vi "Get Menu Bottom Position.vi"(8 "error in (no error)":errorcluster, 11 "MenuButton in":refnum<class "MenuButton.lvclass">) -> (0 "error out":errorcluster, 2 "Menu Bottom Position":u32, 3 "MenuButton out":refnum<class "MenuButton.lvclass">)   [LabVIEW 2017, in "MenuButtons.lvlib" / "MenuButton.lvclass"]
uses:
  MenuButton.lvclass
  MenuButton.lvclass/MenuButton.ctl
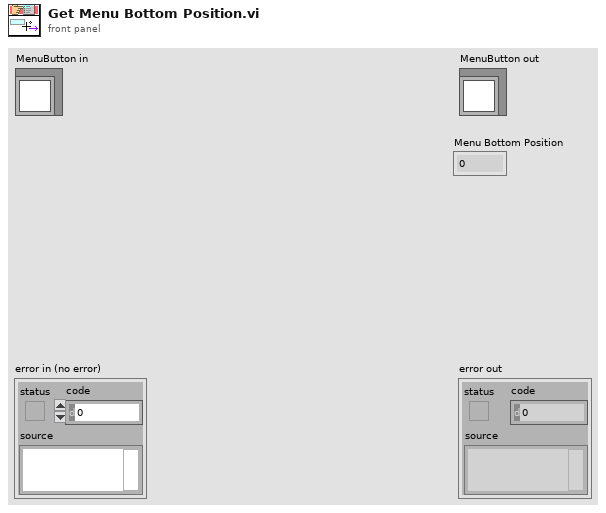
[diagram p1: front panel]
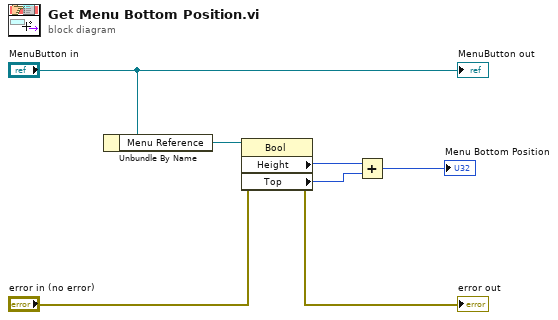
[diagram p0: block diagram]
diagram:
  n1 = Unbundle By Name("MenuButton in") -> ("Menu Reference"=w4:refnum<vi>)
  n2 = property class="Bool"(reference=w4, error in="error in (no error)") -> (error out=→"error out":errorcluster, "Height"=w3:u32, "Top"=w2:i32)  [unwired: 1 out]
  n3 = Add(x=w3, y=w2) -> (x+y=→"Menu Bottom Position":u32)
  "MenuButton out" <- "MenuButton in"
